vi "set_hardware.vi"(8 "error in (no error)":errorcluster, 10 "new_hardware":refnum<class "Hardware.lvclass">, 11 "Measurement in":refnum<class "Measurement.lvclass">) -> (0 "error out":errorcluster, 3 "Measurement out":refnum<class "Measurement.lvclass">)   [LabVIEW 2017, in "Measurement.lvclass"]
doc: "Change the hardware used in the measurement."
uses:
  Measurement.lvclass
  hardware/Hardware.lvclass
  Measurement.lvclass/Measurement.ctl
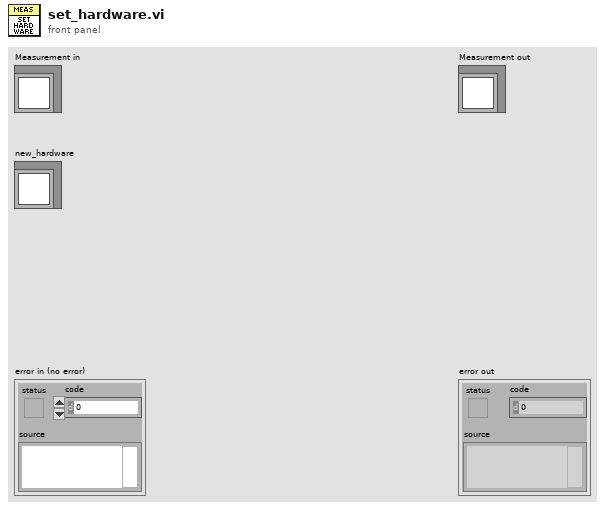
[diagram p1: front panel]
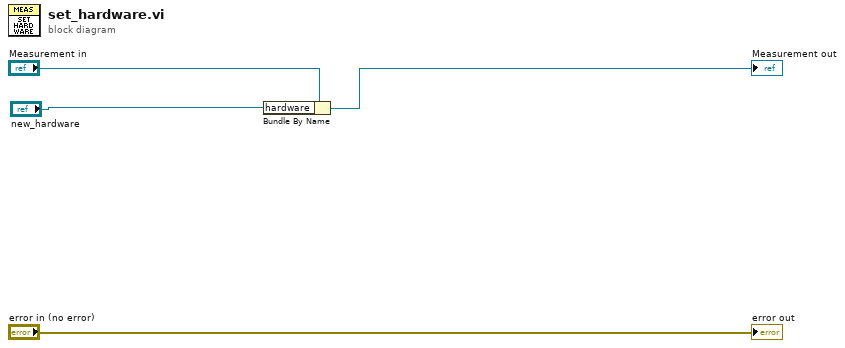
[diagram p0: block diagram]
diagram:
  n1 = Bundle By Name(cluster="Measurement in", "hardware"="new_hardware") -> (→"Measurement out":refnum<class "Measurement.lvclass">)
  "error out" <- "error in (no error)"
